vi "Min_max_pend.vi"(8 "PendEncValMax":u16, 9 "PendEncValMin":u16, 11 "Pendulum Enc":u16) -> (0 "PendEncValMax 2":u16, 3 "PendEncValMin 2":u16)   [LabVIEW 2022 SP3]
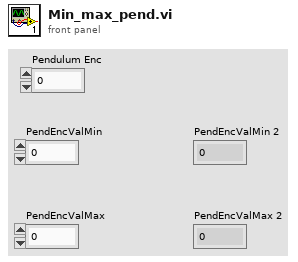
[diagram p1: front panel]
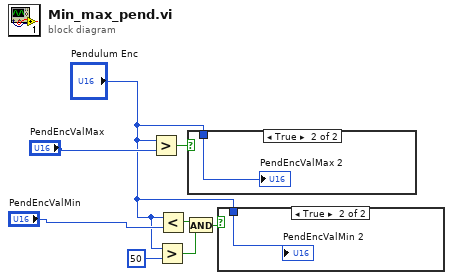
[diagram p0: block diagram]
diagram:
  n1 = Greater?(x="Pendulum Enc", y="PendEncValMax") -> (0:w8:bool)
  n2 = Greater?(x="Pendulum Enc", y=u16 50) -> (0:w4:bool)
  n3 = Less?(x="Pendulum Enc", y="PendEncValMin") -> (x < y?=w5:bool)
  n4 = And(x=w5, y=w4) -> (x .and. y?=w6:bool)
  n5 = case shown="True" w8 {
    tunnel: "Pendulum Enc" -> [_ w9]
    frame False {
    }
    frame True {
      "PendEncValMax 2" <- w9
    }
  }
  n6 = case shown="True" w6 {
    tunnel: "Pendulum Enc" -> [_ w10]
    frame False {
    }
    frame True {
      "PendEncValMin 2" <- w10
    }
  }
